vi "Get Modal VIs.vi"(8 "error in":errorcluster, 11 "Application in":refnum<vi>) -> (0 "error out":errorcluster, 2 "Modal VIs":string[](array[string]), 3 "Application out":refnum<vi>)   [LabVIEW 2013, in "LVTM.lvlib"]
uses:
  LVTM.lvlib
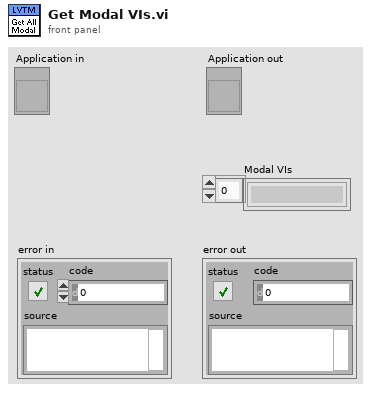
[diagram p1: front panel]
types:
  T1 = enum32{"Invalid", "Default", "Floating", "Floating/Auto-Hide", "Modal"}
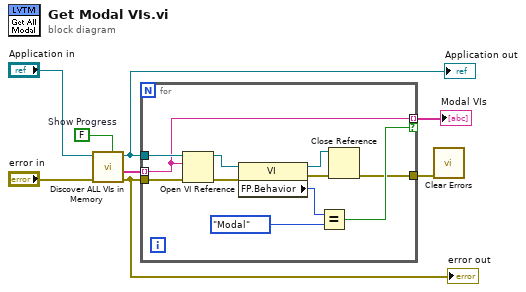
[diagram p0: block diagram]
diagram:
  w1 = FALSE  # Show Progress
  n1 = call "Discover ALL VIs in Memory.vi"("Show Progress (T)"=w1, "error in"="error in", "Application in"="Application in") -> ("error out"=w3:errorcluster, "VIs (including clones)"=w6:string[], "Application out"=w2:refnum<vi>)  [unwired: 6 in]
  "error out" <- w3
  "Application out" <- w2
  n2 = for {
    tunnel: w2 -> [w15]
    tunnel: w3 -> [w14]
    tunnel: w6 -> [w11] mode=indexing
    tunnel: [w11] -> w5 mode=indexing if=w10
    tunnel: [w9] -> w4
    n3 = Open VI Reference(application reference (local)=w15, vi path=w11, error in (no error)=w14) -> (vi reference=w17:refnum<vi>, error out=w16:errorcluster)  [unwired: 3 in]
    n4 = property class="VI"(reference=w17, error in=w16) -> (reference out=w18:refnum<vi>, error out=w19:errorcluster, "FP.Behavior"=w13:T1)
    n5 = Equal?(x=w13, y=T1."Modal" ("Front Panel Window:Behavior")) -> (x = y?=w10:bool)
    n6 = Close Reference(reference=w18, error in (no error)=w19) -> (error out=w9:errorcluster)
  }
  "Modal VIs" <- w5
  n7 = call <vilib>:"Clear Errors.vi"("error in (no error)"=w4) -> ()  [unwired: 6 in, 1 out]
